vi "Get Synapses per Neuron.vi"() -> (0 "Post Neurons Array":cluster{string, i32[]}[](array[cluster]))   [LabVIEW 2016]
doc: "This vi generates an array containing per each Neuron the indexes of the synaptic connections where the neuron is a target (post synaptic euron)"
uses:
  Controls/Type of Synapses.ctl
  Controls/Type of Neuron.ctl
panel:
  out "dummy":T1
  out "dummy2":T2=enum."BA"
  in  "Type of Neuron":T2=enum."BA"
  in  "Synapse":T1
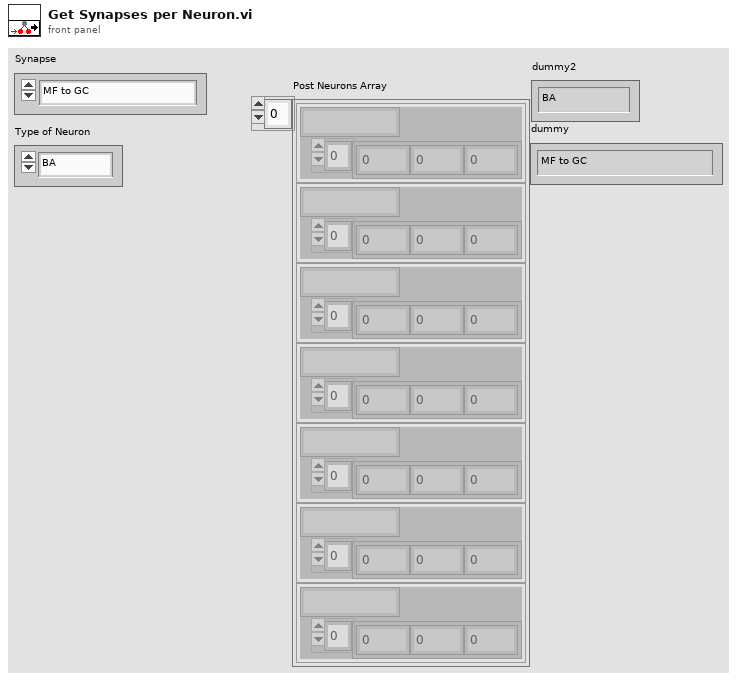
[diagram p1: front panel]
types:
  T1 = typedef "Type of Synapses.ctl" = enum16{"MF to GC", "GO to GC", "GC to GO", "MF to GO", "GC to PC", "GC to BA", "PC to BA", "BA to PC", "BA to GO"}
  T2 = typedef "Type of Neuron.ctl" = enum16{"MF", "BA", "GO", "GC", "PC", "LU", "Glia (Dummy)"}
  T3 = cluster{"Neuron":string, "Index Synapses":i32[]}[]
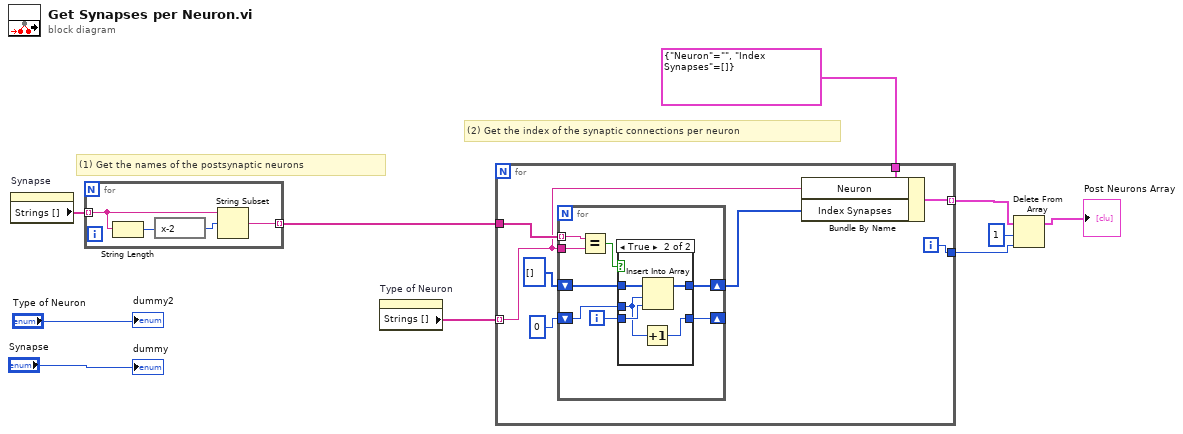
[diagram p0: block diagram]
diagram:
  # "(2) Get the index of the synaptic connections per neuron"
  # "(1) Get the names of the postsynaptic neurons"
  n1 = property on="Synapse" class="Enum (strict)"() -> ("Strings []"=w10:string[])  [unwired: 2 in, 2 out]
  n2 = for {
    tunnel: w10 -> [w14] mode=indexing
    tunnel: [w11] -> w8 mode=indexing
    n3 = String Length(string=w14) -> (length=w13:i32)
    n4 = expression code="x-2"(w13) -> (w12:i32)
    n5 = String Subset(string=w14, offset (0)=w12) -> (substring=w11:string)  [unwired: 1 in]
  }
  n6 = property on="Type of Neuron" class="Enum (strict)"() -> ("Strings []"=w9:string[])  [unwired: 2 in, 2 out]
  n7 = for {
    tunnel: w9 -> [w19] mode=indexing
    tunnel: w8 -> [w22]
    tunnel: [w17] -> w6 mode=indexing
    tunnel: cluster{"Neuron":string, "Index Synapses":i32[]} {"Neuron"="", "Index Synapses"=[]} -> [w16]
    tunnel: [w15] -> w3
    i -> [w15]
    n8 = for {
      tunnel: w22 -> [w30] mode=indexing
      tunnel: w19 -> [w29]
      shift-right: [w23] -> _
      shift-left: 0 -> [w27]
      shift-right: [w24] -> w18
      shift-left: i32[] [] -> [w25]
      i -> [w28]
      n9 = Equal?(x=w30, y=w29) -> (x = y?=w26:bool)
      n10 = case shown="True" w26 {
        tunnel: w28 -> [_ w37]
        tunnel: w27 -> [w31 w34]
        tunnel: w25 -> [w32 w36]
        tunnel: [w32 w35] -> w24
        tunnel: [w31 w33] -> w23
        frame False {
        }
        frame True {
          n11 = Increment(x=w34) -> (x+1=w33:i32)
          n12 = Insert Into Array(array=w36, index=w34, new element=w37) -> (w35:i32[])
        }
      }
    }
    n13 = Bundle By Name(cluster=w16, "Neuron"=w19, "Index Synapses"=w18) -> (w17:cluster{"Neuron":string, "Index Synapses":i32[]})
  }
  n14 = Delete From Array(array=w6, length=1, index=w3) -> (array with subset deleted=→"Post Neurons Array":T3)  [unwired: 1 out]
  "dummy2" <- "Type of Neuron"
  "dummy" <- "Synapse"
